vi "sava-4.vi"(7 "datafile":path[](array[path]), 8 "1D array 4":i16[](array[numeric]) caption="一维数组-4", 9 "1D array 3":i16[](array[numeric]) caption="一维数组-3", 10 "1D array 2":i16[](array[numeric]) caption="一维数组-2", 11 "1D array":i16[](array[numeric]) caption="一维数组-1") -> ()   [LabVIEW 2012]
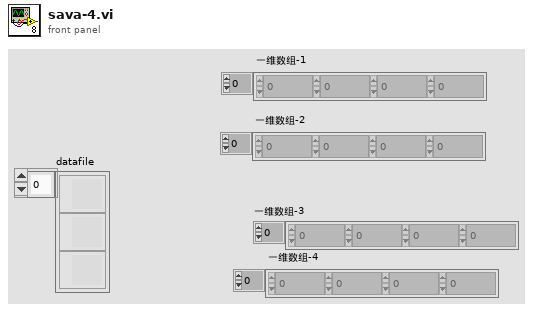
[diagram p1: front panel]
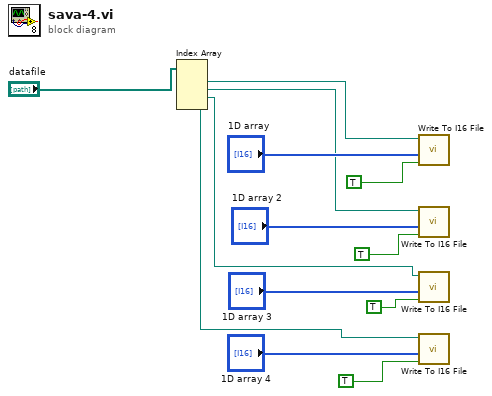
[diagram p0: block diagram]
diagram:
  n1 = Index Array(array="datafile") -> (element #1=w4:path, element #2=w3:path, element #3=w2:path, element #4=w1:path)  [unwired: 4 in]
  n2 = call <vilib>:"Write To I16 File.vi"("append to file? (new file:F)"=TRUE, "1D array"="1D array", "file path (dialog if empty)"=w4) -> ()  [unwired: 4 in, 1 out]
  n3 = call <vilib>:"Write To I16 File.vi"("append to file? (new file:F)"=TRUE, "1D array"="1D array 2", "file path (dialog if empty)"=w3) -> ()  [unwired: 4 in, 1 out]
  n4 = call <vilib>:"Write To I16 File.vi"("append to file? (new file:F)"=TRUE, "1D array"="1D array 3", "file path (dialog if empty)"=w2) -> ()  [unwired: 4 in, 1 out]
  n5 = call <vilib>:"Write To I16 File.vi"("append to file? (new file:F)"=TRUE, "1D array"="1D array 4", "file path (dialog if empty)"=w1) -> ()  [unwired: 4 in, 1 out]
